vi "getDescription.vi"(8 "error in (no error)":errorcluster, 10 "test":refnum<class>, 11 "TestTestResult in":refnum<class "_TextTestResult.lvclass">) -> (0 "error out":errorcluster, 2 "description":string, 3 "TestTestResult in":refnum<class "_TextTestResult.lvclass">)   [LabVIEW 2011, in "_TextTestResult.lvclass"]
uses:
  _TextTestResult.lvclass
  TestCase/TestCase.lvclass
  _TextTestResult.lvclass/_TextTestResult.ctl
  TestSuite/TestSuite.lvclass
panel:
  # "JKI VI Tester for LabVIEW\nhttp://jkisoft.com/vi-tester\nCopyright (C) 2007-2009, JKI <info@jkisoft.com>\nALL RIGHTS RESERVED"
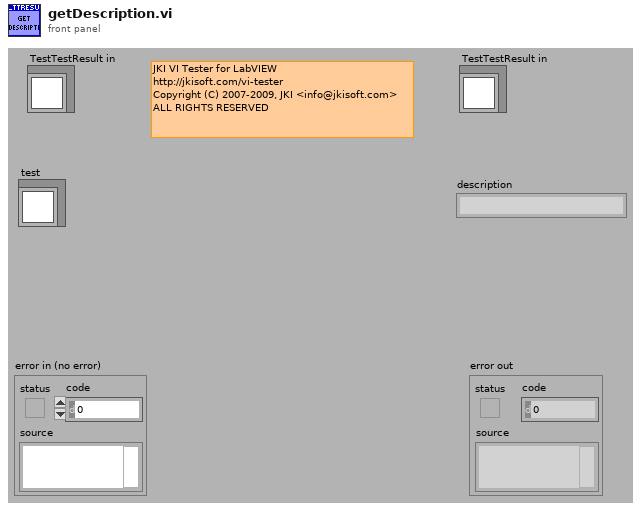
[diagram p1: front panel]
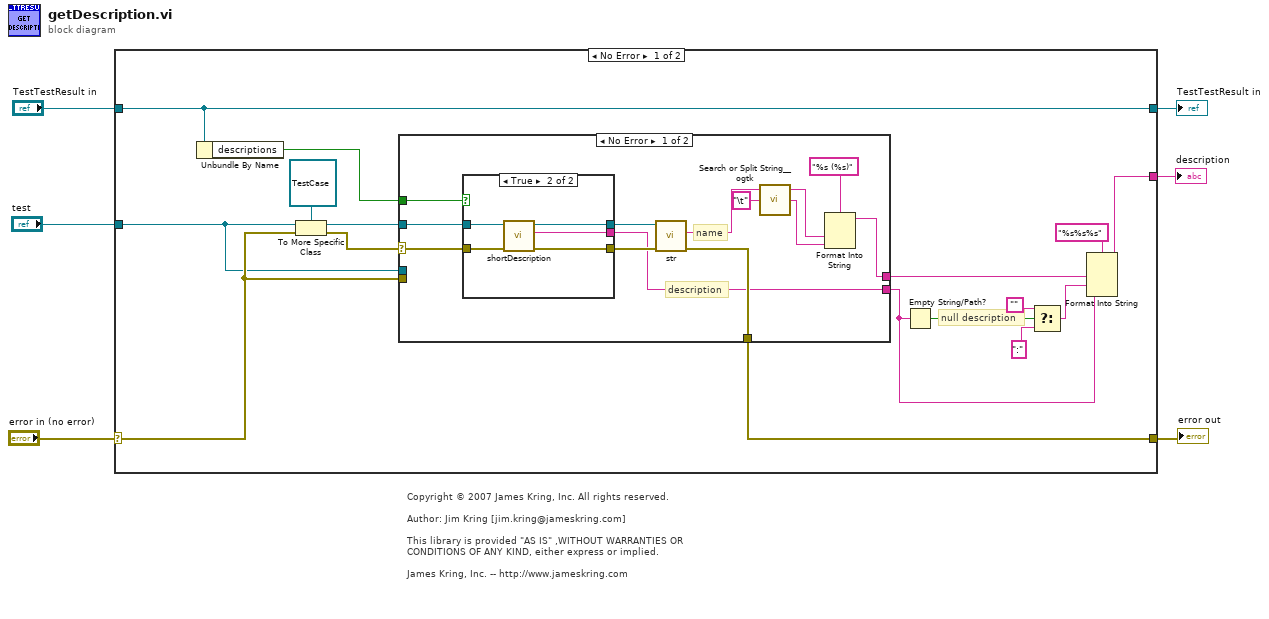
[diagram p0: block diagram]
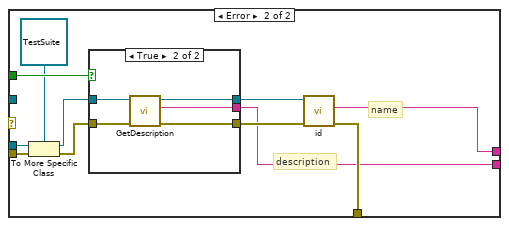
[diagram p3: hidden frame]
diagram:
  # "Copyright © 2007 James Kring, Inc. All rights reserved.\n\nAuthor: Jim Kring [jim.kring@jameskring.com]\n\nThis library is provided \"AS IS\" ,WITHOUT WARRANTIES OR \nCONDITIONS OF ANY KIND, either express or implied.\n\nJames Kring, Inc. -- http://www.jameskring.com"
  n1 = case shown="No Error" "error in (no error)" {
    selector: "error in (no error)" -> [w16 w62]
    tunnel: [w17 w62] -> w5
    tunnel: [w22 w61] -> w3
    tunnel: "TestTestResult in" -> [w22 w61]
    tunnel: "test" -> [w15 _]
    tunnel: [w13 _] -> w1
    frame No Error {
      # "null description"
      n2 = Unbundle By Name(w22) -> ("descriptions"=w18:bool)
      n3 = To More Specific Class(target class=refnum<class "TestCase.lvclass"> refnum ("reference in"), reference=w15, error in=w16) -> (specific class reference=w20:refnum<class "TestCase.lvclass">, error out=w19:errorcluster)
      n4 = case shown="No Error" w19 {
        selector: w19 -> [w30 _]
        tunnel: w20 -> [w35 _]
        tunnel: w18 -> [w34 w53]
        tunnel: [w32 w51] -> w17
        tunnel: w16 -> [_ w49]
        tunnel: w15 -> [_ w47]
        tunnel: [w23 w44] -> w14
        tunnel: [w29 w43] -> w7
        frame No Error {
          # "name"
          # "description"
          n5 = case shown="True" w34 {
            tunnel: [w37 w42] -> w31
            tunnel: [_ w41] -> w29
            tunnel: w35 -> [w36 w40]
            tunnel: w30 -> [w37 w39]
            tunnel: [w36 w38] -> w33
            frame False {
            }
            frame True {
              n6 = call-dynamic "shortDescription.vi"("error in (no error)"=w39, "TestCase in"=w40) -> ("error out"=w42:errorcluster, "description"=w41:string, "TestCase out"=w38:refnum<class "TestCase.lvclass">)  [unwired: 7 in]
            }
          }
          n7 = call-dynamic "str.vi"("error in (no error)"=w31, "TestCase in"=w33) -> ("error out"=w32:errorcluster, "string"=w24:string)  [unwired: 7 in, 1 out]
          n8 = call <userlib>:"Search or Split String__ogtk.vi"("search string/char (-)"="\t", "string"=w24) -> ("substring after match"=w26:string, "substring before match"=w27:string)  [unwired: 1 in, 1 out]
          n9 = Format Into String(format string="%s (%s)", w27, w26) -> (resulting string=w23:string)  [unwired: 2 in, 1 out]
        }
        frame Error {
          # "description"
          # "name"
          n10 = To More Specific Class(target class=refnum<class "TestSuite.lvclass"> refnum ("reference in"), reference=w47, error in=w49) -> (specific class reference=w45:refnum<class "TestSuite.lvclass">, error out=w46:errorcluster)
          n11 = case shown="True" w53 {
            tunnel: [w55 w60] -> w50
            tunnel: [_ w59] -> w43
            tunnel: w45 -> [w54 w58]
            tunnel: w46 -> [w55 w57]
            tunnel: [w54 w56] -> w52
            frame False {
            }
            frame True {
              n12 = call-dynamic "GetDescription.vi"("error in (no error)"=w57, "TestSuite in"=w58) -> ("error out"=w60:errorcluster, "Description"=w59:string, "TestSuite out"=w56:refnum<class "TestSuite.lvclass">)  [unwired: 7 in]
            }
          }
          n13 = call-dynamic "id.vi"("error in (no error)"=w50, "TestSuite in"=w52) -> ("error out"=w51:errorcluster, "Description"=w44:string)  [unwired: 6 in, 2 out]
        }
      }
      n14 = Empty String/Path?(string/path=w7) -> (empty?=w11:bool)
      n15 = Select(t="", s=w11, f=":" ("format string")) -> (s? t:f=w8:string)
      n16 = Format Into String(format string="%s%s%s", w14, w8, w7) -> (resulting string=w13:string)  [unwired: 2 in, 1 out]
    }
    frame Error {
    }
  }
  "error out" <- w5
  "TestTestResult in" <- w3
  "description" <- w1
